vi "DSC TSV Process Files with Queues.vi"(7 "reference":refnum<vi>, 8 "error in":errorcluster, 9 "File Path":path, 10 "variable":string, 11 "Data.PG in":refnum<class "LV-Data.PGSQL.lvclass">) -> (0 "error out":errorcluster)   [LabVIEW 2019]
uses:
  src/LV-Data.PG/LV-Data.PGSQL.lvclass
  src/LV-Data.PG/Private/INSERT Multivalue.vi
panel:
  out "array of clusters":cluster{"String":string}[](array[cluster])
  out "Array":timestamp[](array[timestamp])
  out "Numeric":i32
  out "Iteration terminal":i32
  in  "Stop":bool
  in  "Number of row to read \nat a time":i32=10000
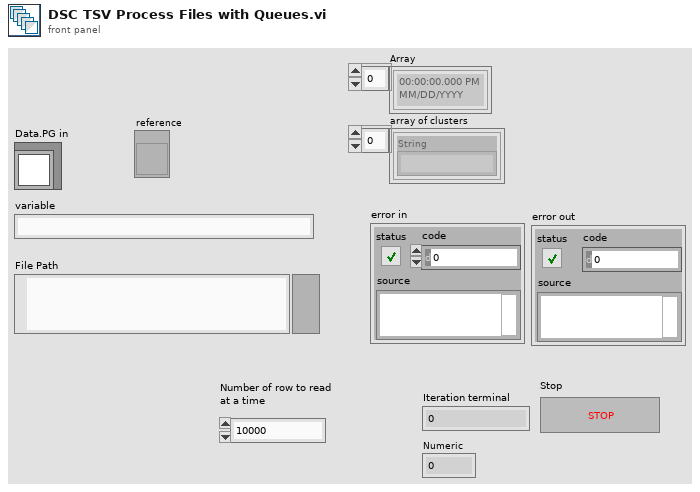
[diagram p1: front panel]
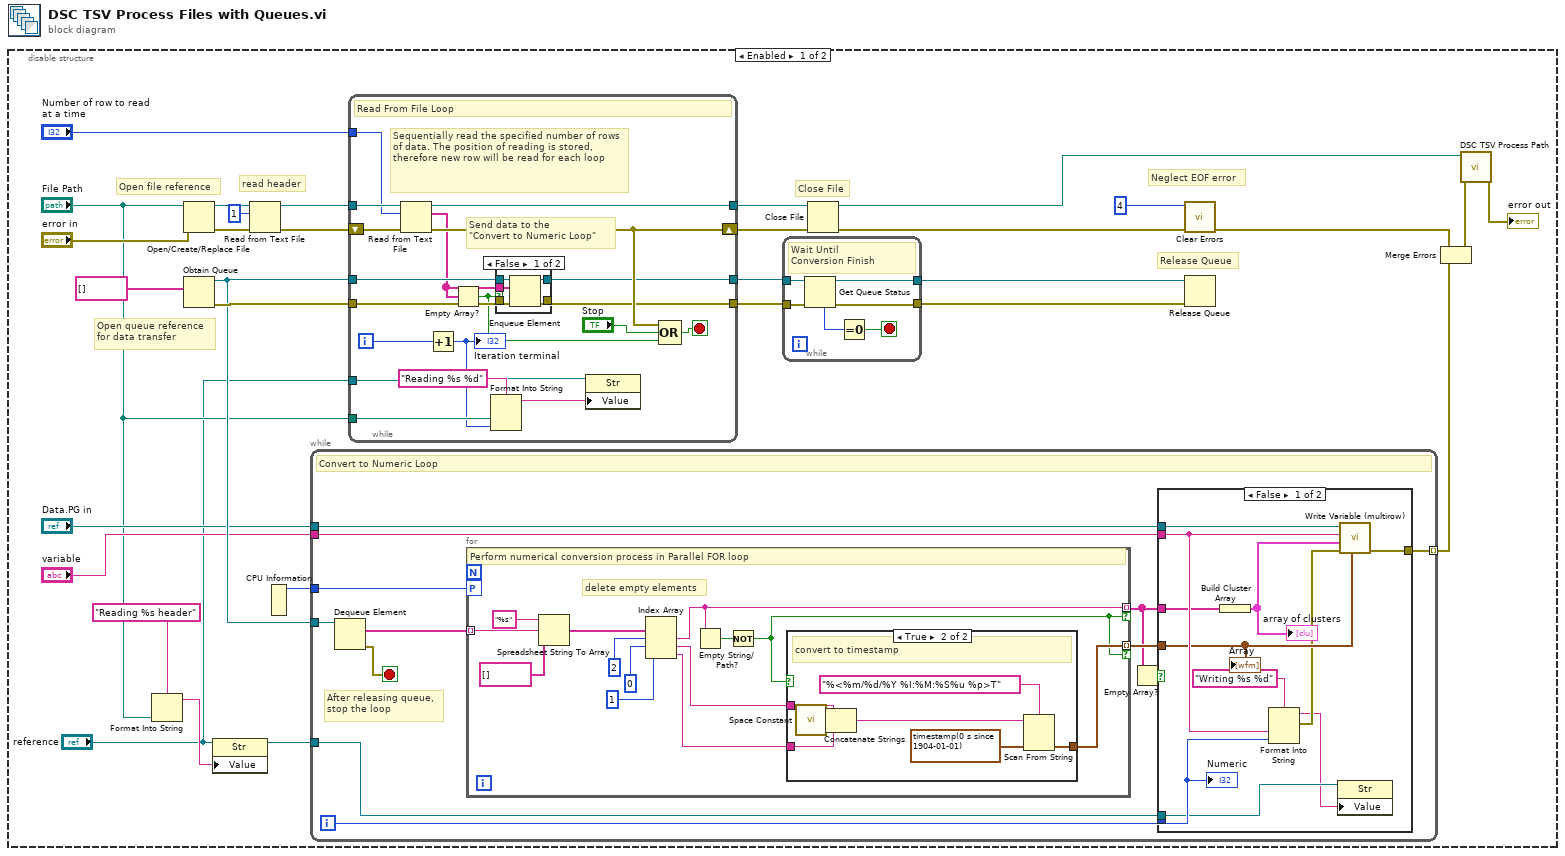
[diagram p0: block diagram]
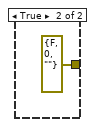
[diagram p2: hidden frame]
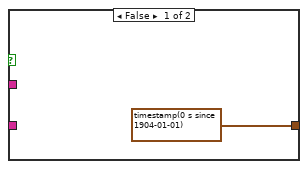
[diagram p3: hidden frame]
diagram:
  n1 = disable-structure shown="Enabled" {
    frame Enabled {
      # "read header"
      # "Neglect EOF error"
      # "Release Queue"
      # "Close File"
      # "Open queue reference\nfor data transfer"
      # "Open file reference"
      n2 = Format Into String(format string="Reading %s header", "File Path") -> (resulting string=w5:string)  [unwired: 2 in, 1 out]
      n3 = Open/Create/Replace File(file path (use dialog)="File Path", error in="error in") -> (refnum out=w19:refnum<file>, error out=w16:errorcluster)  [unwired: 4 in, 1 out]
      n4 = Obtain Queue(element data type=string[] [] ("形式文字列")) -> (queue out=w24:refnum<queue>, error out=w25:errorcluster)  [unwired: 4 in, 1 out]
      n5 = property class="Str"(reference="reference", "Value"=w5) -> (reference out=w2:refnum<vi>)  [unwired: 1 in, 1 out]
      n6 = Read from Text File(file (use dialog)=w19, count=1, error in=w16) -> (refnum out=w18:refnum<file>, error out=w17:errorcluster)  [unwired: 1 in, 2 out]
      n7 = CPU Information() -> (4:w1:i32)  [unwired: 3 out]
      n8 = while {
        tunnel: w24 -> [w43]
        tunnel: "Data.PG in" -> [w41]
        tunnel: "variable" -> [w39]
        tunnel: [w40] -> w11 mode=indexing
        tunnel: w2 -> [w37]
        tunnel: w1 -> [w34]
        i -> [w38]
        stop <- w42 stop-if-true
        # "After releasing queue,\nstop the loop"
        # "Convert to Numeric Loop"
        n9 = Dequeue Element(queue=w43) -> (element=w36:string[], error out=w42:errorcluster)  [unwired: 2 in, 2 out]
        n10 = for "Forループ" {
          workers-P: w34 -> [_]
          tunnel: w36 -> [w66] mode=indexing
          tunnel: [w56] -> w33 mode=indexing if=w57
          tunnel: [w58] -> w35 mode=indexing if=w57
          # "delete empty elements"
          # "Perform numerical conversion process in Parallel FOR loop"
          n11 = Spreadsheet String To Array(format string="%s", spreadsheet string=w66, array type (2D Dbl)=string[] []) -> (array=w65:string[])  [unwired: 1 in]
          n12 = Index Array(array=w65, index #1=2 ("disabled index (col)"), index #2=0 ("disabled index (col)"), index #3=1 ("disabled index (col)")) -> (element #1=w56:string, element #2=w60:string, element #3=w59:string)
          n13 = Empty String/Path?(string/path=w56) -> (empty?=w61:bool)
          n14 = Not(x=w61) -> (.not. x?=w57:bool)
          n15 = case shown="True" w57 {
            tunnel: w60 -> [_ w70]
            tunnel: w59 -> [_ w71]
            tunnel: [timestamp(0 s since 1904-01-01) ("default value 1") w72] -> w58
            frame False {
            }
            frame True {
              # "convert to timestamp"
              n16 = call <vilib>:"Space Constant.vi"() -> ("String"=w76:string)
              n17 = Concatenate Strings(w70, w76, w71) -> (w73:string)
              n18 = Scan From String(format string="%<%m/%d/%Y %I:%M:%S%u %p>T", input string=w73, default 1=timestamp(0 s since 1904-01-01) ("default value 1")) -> (output 1=w72:timestamp)  [unwired: 2 in, 3 out]
            }
          }
        }
        n19 = Empty Array?(array=w33) -> (empty?=w32:bool)
        n20 = case shown="False" w32 {
          tunnel: w41 -> [w54 _]
          tunnel: [w53 errorcluster {"status"=FALSE, "code"=0, "source"=""} ("error out")] -> w40
          tunnel: w39 -> [w52 _]
          tunnel: w38 -> [w51 _]
          tunnel: w37 -> [w50 _]
          tunnel: w35 -> [w49 _]
          tunnel: w33 -> [w44 _]
          frame False {
            n21 = Build Cluster Array(w44) -> (w45:cluster{"String":string}[])
            "array of clusters" <- w45
            n22 = Format Into String(format string="Writing %s %d", w52, w51) -> (resulting string=w46:string, error out=w47:errorcluster)  [unwired: 2 in]
            n23 = property class="Str"(reference=w50, "Value"=w46) -> ()  [unwired: 1 in, 2 out]
            n24 = call "Write Variable (multirow).vi"("Time Stamps"=w49, "error in (no error)"=w47, "Data"=w45, "Path(s)"=w52, "Data.PG in"=w54) -> ("error out"=w53:errorcluster)  [unwired: 3 in, 3 out]
            "Numeric" <- w51
            "Array" <- w49
          }
          frame True {
          }
        }
      }
      n25 = while {
        tunnel: w18 -> [w101]
        tunnel: [w99] -> w31
        shift-right: [w95] -> w30
        shift-left: w17 -> [w100]
        tunnel: "Number of row to read \nat a time" -> [w96]
        tunnel: w24 -> [w94]
        tunnel: w25 -> [w93]
        tunnel: [w92] -> w23
        tunnel: [w91] -> w22
        tunnel: "File Path" -> [w89]
        tunnel: "reference" -> [w86]
        i -> [w97]
        stop <- w98 stop-if-true
        # "Send data to the \n\"Convert to Numeric Loop\""
        # "Sequentially read the specified number of rows of data. The position of reading is stored, therefore new row will be read for each loop"
        # "Read From File Loop"
        n26 = Read from Text File(file (use dialog)=w101, count=w96, error in=w100) -> (refnum out=w99:refnum<file>, text=w85:string[], error out=w95:errorcluster)  [unwired: 1 in, 1 out]
        n27 = Increment(x=w97) -> (x+1=w88:i32)
        "Iteration terminal" <- w88
        n28 = Empty Array?(array=w85) -> (empty?=w83:bool)
        n29 = Format Into String(format string="Reading %s %d", w89, w88) -> (resulting string=w87:string)  [unwired: 2 in, 1 out]
        n30 = case shown="False" w83 {
          tunnel: w94 -> [w106 w108]
          tunnel: w93 -> [w105 w107]
          tunnel: [w104 w108] -> w92
          tunnel: [w103 w107] -> w91
          tunnel: w85 -> [w102 _]
          frame False {
            n31 = Enqueue Element(queue=w106, element=w102, error in (no error)=w105) -> (queue out=w104:refnum<queue>, error out=w103:errorcluster)  [unwired: 1 in, 1 out]
          }
          frame True {
          }
        }
        n32 = property class="Str"(reference=w86, "Value"=w87) -> ()  [unwired: 1 in, 2 out]
        n33 = Compound Arithmetic op=OR(w95, "Stop", w83) -> (w98:bool)
      }
      n34 = while {
        tunnel: w23 -> [w82]
        tunnel: w22 -> [w81]
        tunnel: [w78] -> w20
        tunnel: [w77] -> w21
        stop <- w79 stop-if-true
        # "Wait Until \nConversion Finish"
        n35 = Get Queue Status(queue=w82, error in (no error)=w81) -> (queue out=w78:refnum<queue>, error out=w77:errorcluster, # elements in queue=w80:i32)  [unwired: 1 in, 5 out]
        n36 = Equal To 0?(x=w80) -> (x = 0?=w79:bool)
      }
      n37 = Close File(refnum=w31, error in=w30) -> (path=w7:path, error out=w29:errorcluster)
      n38 = call <vilib>:"Clear Errors.vi"("error in (no error)"=w29, "specific error code to clear (0: all)"=4) -> ("error out"=w9:errorcluster)  [unwired: 4 in, 1 out]
      n39 = Release Queue(queue=w20, error in (no error)=w21) -> ()  [unwired: 1 in, 3 out]
      n40 = Merge Errors(w9, w11) -> (w10:errorcluster)
      n41 = call "DSC TSV Process Path.vi"("error in (no error)"=w10, "path in"=w7) -> ("error out"=→"error out":errorcluster)  [unwired: 7 in, 2 out]
    }
    frame Disabled {
    }
  }
